vi "Get Current Point.vi"(0 "eye scan point iterator":refnum<class "niHighSpeedSerial N Point Eye Scan Point Iterator v1 Host.lvclass">, 11 "error in":errorcluster) -> (4 "eye scan point iterator out":refnum<class "niHighSpeedSerial N Point Eye Scan Point Iterator v1 Host.lvclass">, 6 "current point":T1, 15 "error out":errorcluster)   [LabVIEW 2014, in "niHighSpeedSerial N Point Eye Scan Point Iterator v1 Host.lvclass"]
doc: "Returns the point currently being measured.\n\n<B>Input Parameters</B>\n\n<B>eye scan point iterator</B> is the incoming wire for the Eye Scan Point Iterator class object\n\n<B>error in</B> describes error conditions that occur before this node runs. This input provides standard 'error in' functionality.\n\n<B>Output Parameters</B>\n\n<B>eye scan point iterator out</B> is the outgoing wire for the Eye Scan Point Iterator class object\n\n<B>current point</B> is the point currently being measured.\n\n<B>current point.horizontal offset</B> is the horizontal offset of the point currently being measured.\n\n<B>current point.vertical offset</B> is the vertical offset of the point currently being measured.\n\n<B>error out</B> contains error information. This output provides standard 'error out' functionality."
uses:
  <instrlib>/niHighSpeedSerial/Eye Scan/v1/Host/Impl/N Pt Iter/niHighSpeedSerial N Point Eye Scan Point Iterator v1 Host.lvclass
  <instrlib>/niHighSpeedSerial/Eye Scan/v1/Host/Common/Public/Point Offsets.ctl
  <instrlib>/niHighSpeedSerial/Eye Scan/v1/Host/Impl/N Pt Iter/niHighSpeedSerial N Point Eye Scan Point Iterator v1 Host.lvclass/niHighSpeedSerial N Point Eye Scan Point Iterator v1 Host.ctl
  <instrlib>/niHighSpeedSerial/Eye Scan/v1/Host/Common/niHighSpeedSerial Eye Scan Common v1 Host.lvlib
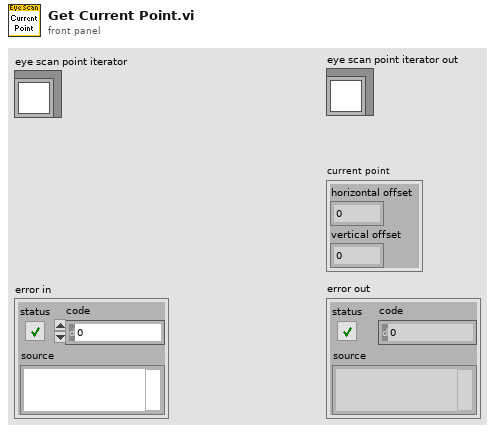
[diagram p1: front panel]
types:
  T1 = typedef "niHighSpeedSerial Eye Scan Common v1 Host.lvlib/Point Offsets.ctl" = cluster{"horizontal offset":i16, "vertical offset":i8}
  T2 = typedef "niHighSpeedSerial Eye Scan Common v1 Host.lvlib/Point.ctl" = cluster{"point offsets":T1, "sample count":u64, "error count":u64, "bit error rate":dbl}
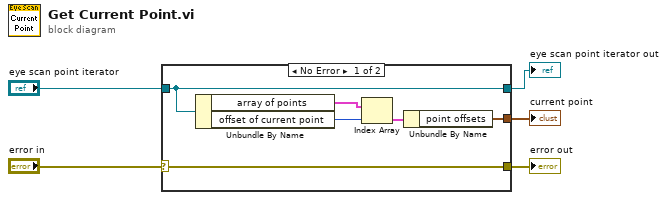
[diagram p0: block diagram]
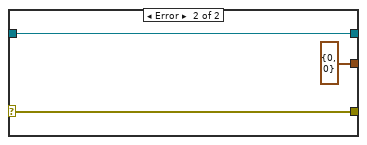
[diagram p2: hidden frame]
diagram:
  n1 = case shown="No Error" "error in" {
    selector: "error in" -> [w11 w14]
    tunnel: "eye scan point iterator" -> [w6 w13]
    tunnel: [w11 w14] -> w3
    tunnel: [w6 w13] -> w2
    tunnel: [w10 T1 {"horizontal offset"=0, "vertical offset"=0} ("Current Point")] -> w1
    frame No Error {
      n2 = Unbundle By Name(w6) -> ("array of points"=w9:T2[], "offset of current point"=w8:i32)
      n3 = Index Array(array=w9, index=w8) -> (element=w7:T2)
      n4 = Unbundle By Name(w7) -> ("point offsets"=w10:T1)
    }
    frame Error {
    }
  }
  "eye scan point iterator out" <- w2
  "error out" <- w3
  "current point" <- w1
